vi "加载默认参数.vi"(11 "error IO":errorcluster) -> ()   [LabVIEW 2016, in "环境动力监测库.lvlib"]
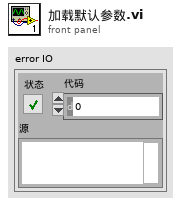
[diagram p1: front panel]
types:
  T1 = cluster{"功能启用":bool, "排气扇开启温度":dbl, "排气扇关闭温度":dbl}
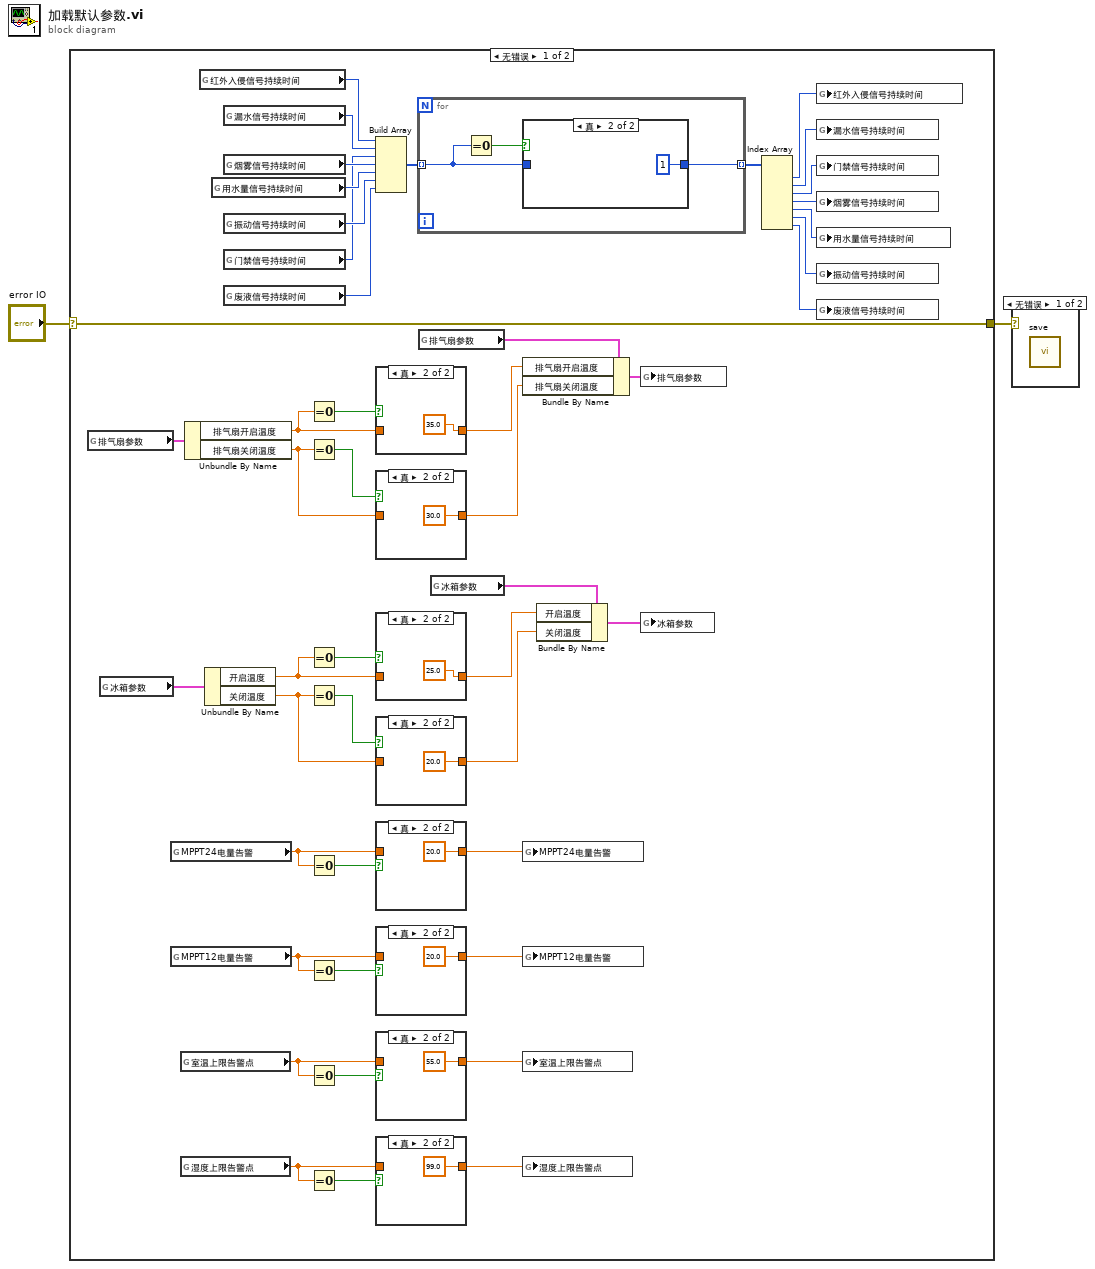
[diagram p0: block diagram]
diagram:
  n1 = case shown="无错误" "error IO" {
    selector: "error IO" -> [w40 w71]
    tunnel: [w40 w71] -> w2
    frame No Error {
      n2 = global read "断电保存全局变量.vi" "排气扇参数"() -> (w49:T1)
      n3 = global read "断电保存全局变量.vi" "冰箱参数"() -> (w3:cluster{"功能启用":bool, "开启温度":dbl, "关闭温度":dbl})
      n4 = global read "断电保存全局变量.vi" "MPPT24电量告警"() -> (w16:dbl)
      n5 = global read "断电保存全局变量.vi" "MPPT12电量告警"() -> (w17:dbl)
      n6 = global read "断电保存全局变量.vi" "室温上限告警点"() -> (w35:dbl)
      n7 = global read "断电保存全局变量.vi" "湿度上限告警点"() -> (w34:dbl)
      n8 = Unbundle By Name(w49) -> ("排气扇开启温度"=w43:dbl, "排气扇关闭温度"=w41:dbl)
      n9 = global read "断电保存全局变量.vi" "红外入侵信号持续时间"() -> (w18:u32)
      n10 = Unbundle By Name(w3) -> ("开启温度"=w9:dbl, "关闭温度"=w11:dbl)
      n11 = global read "断电保存全局变量.vi" "用水量信号持续时间"() -> (w22:u32)
      n12 = global read "断电保存全局变量.vi" "漏水信号持续时间"() -> (w19:u32)
      n13 = global read "断电保存全局变量.vi" "烟雾信号持续时间"() -> (w21:u32)
      n14 = global read "断电保存全局变量.vi" "振动信号持续时间"() -> (w23:u32)
      n15 = global read "断电保存全局变量.vi" "门禁信号持续时间"() -> (w20:u32)
      n16 = global read "断电保存全局变量.vi" "废液信号持续时间"() -> (w24:u32)
      n17 = Equal To 0?(x=w43) -> (x = 0?=w44:bool)
      n18 = Equal To 0?(x=w41) -> (x = 0?=w42:bool)
      n19 = Equal To 0?(x=w9) -> (x = 0?=w8:bool)
      n20 = Equal To 0?(x=w11) -> (x = 0?=w10:bool)
      n21 = Equal To 0?(x=w16) -> (x = 0?=w14:bool)
      n22 = Equal To 0?(x=w17) -> (x = 0?=w15:bool)
      n23 = Equal To 0?(x=w35) -> (x = 0?=w37:bool)
      n24 = Equal To 0?(x=w34) -> (x = 0?=w36:bool)
      n25 = Build Array(w18, w19, w20, w21, w22, w23, w24) -> (w25:u32[])
      n26 = case shown="真" w44 {
        tunnel: [w69 35.0 ("值(信号)")] -> w46
        tunnel: w43 -> [w69 _]
        frame False {
        }
        frame True {
        }
      }
      n27 = case shown="真" w42 {
        tunnel: [w67 30.0 ("排气扇开启温度")] -> w45
        tunnel: w41 -> [w67 _]
        frame False {
        }
        frame True {
        }
      }
      n28 = case shown="真" w8 {
        tunnel: [w52 25.0 ("值(信号)")] -> w6
        tunnel: w9 -> [w52 _]
        frame False {
        }
        frame True {
        }
      }
      n29 = case shown="真" w10 {
        tunnel: [w50 20.0 ("排气扇开启温度")] -> w7
        tunnel: w11 -> [w50 _]
        frame False {
        }
        frame True {
        }
      }
      n30 = case shown="真" w14 {
        tunnel: [w56 20.0 ("室温上限告警点")] -> w13
        tunnel: w16 -> [w56 _]
        frame False {
        }
        frame True {
        }
      }
      n31 = case shown="真" w15 {
        tunnel: [w54 20.0 ("室温上限告警点")] -> w12
        tunnel: w17 -> [w54 _]
        frame False {
        }
        frame True {
        }
      }
      n32 = case shown="真" w37 {
        tunnel: [w65 55.0 ("室温上限告警点")] -> w38
        tunnel: w35 -> [w65 _]
        frame False {
        }
        frame True {
        }
      }
      n33 = case shown="真" w36 {
        tunnel: [w63 99.0 ("室温上限告警点")] -> w39
        tunnel: w34 -> [w63 _]
        frame False {
        }
        frame True {
        }
      }
      n34 = for {
        tunnel: w25 -> [w58] mode=indexing
        tunnel: [w59] -> w26 mode=indexing
        n35 = Equal To 0?(x=w58) -> (x = 0?=w60:bool)
        n36 = case shown="真" w60 {
          tunnel: [w61 u32 1 ("红外入侵信号持续时间")] -> w59
          tunnel: w58 -> [w61 _]
          frame False {
          }
          frame True {
          }
        }
      }
      n37 = global read "断电保存全局变量.vi" "排气扇参数"() -> (w47:T1)
      n38 = global read "断电保存全局变量.vi" "冰箱参数"() -> (w5:cluster{"功能启用":bool, "开启温度":dbl, "关闭温度":dbl})
      n39 = Bundle By Name(cluster=w47, "排气扇开启温度"=w46, "排气扇关闭温度"=w45) -> (w48:T1)
      n40 = global write "断电保存全局变量.vi" "MPPT24电量告警"(w13) -> ()
      n41 = global write "断电保存全局变量.vi" "MPPT12电量告警"(w12) -> ()
      n42 = global write "断电保存全局变量.vi" "室温上限告警点"(w38) -> ()
      n43 = global write "断电保存全局变量.vi" "湿度上限告警点"(w39) -> ()
      n44 = Bundle By Name(cluster=w5, "开启温度"=w6, "关闭温度"=w7) -> (w4:cluster{"功能启用":bool, "开启温度":dbl, "关闭温度":dbl})
      n45 = global write "断电保存全局变量.vi" "排气扇参数"(w48) -> ()
      n46 = global write "断电保存全局变量.vi" "冰箱参数"(w4) -> ()
      n47 = Index Array(array=w26) -> (element #1=w27:u32, element #2=w28:u32, element #3=w29:u32, element #4=w30:u32, element #5=w31:u32, element #6=w32:u32, element #7=w33:u32)  [unwired: 7 in]
      n48 = global write "断电保存全局变量.vi" "红外入侵信号持续时间"(w27) -> ()
      n49 = global write "断电保存全局变量.vi" "漏水信号持续时间"(w28) -> ()
      n50 = global write "断电保存全局变量.vi" "门禁信号持续时间"(w29) -> ()
      n51 = global write "断电保存全局变量.vi" "烟雾信号持续时间"(w30) -> ()
      n52 = global write "断电保存全局变量.vi" "用水量信号持续时间"(w31) -> ()
      n53 = global write "断电保存全局变量.vi" "振动信号持续时间"(w32) -> ()
      n54 = global write "断电保存全局变量.vi" "废液信号持续时间"(w33) -> ()
    }
    frame Error {
    }
  }
  n55 = case shown="无错误" w2 {
    frame No Error {
      n56 = call "save.vi"() -> ()  [unwired: 11 in, 1 out]
    }
    frame Error {
    }
  }
